vi "Do.vi"(6 "Input":variant, 8 "error in":errorcluster, 9 "Self Enqueuer":refnum<class "Message Enqueuer.lvclass">, 10 "Series Enqueuer":refnum<class "Message Enqueuer.lvclass">, 11 "Sample Watertemp PWM Control in":refnum<class "Sample Watertemp PWM Control.lvclass">) -> (0 "error out":errorcluster, 3 "Sample Watertemp PWM Control out":refnum<class "Sample Watertemp PWM Control.lvclass">)   [LabVIEW 2023, in "Sample Watertemp PWM Control.lvclass"]
uses:
  Sample Watertemp PWM Control.lvclass
  Sample Watertemp PWM Control.lvclass/Sample Watertemp PWM Control.ctl
  Task/Task Base/Task Base.lvclass
  Measure and Stimulus Subsystems/Measure and Stimulus Subsystems.lvclass
  <vilib>/ActorFramework/Message Enqueuer/Message Enqueuer.lvclass
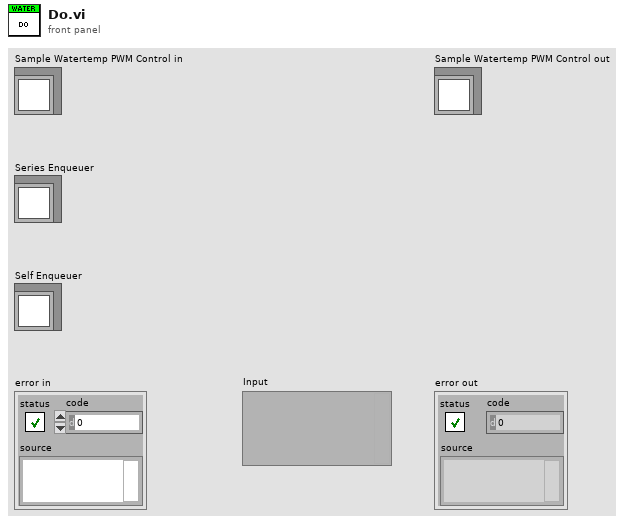
[diagram p1: front panel]
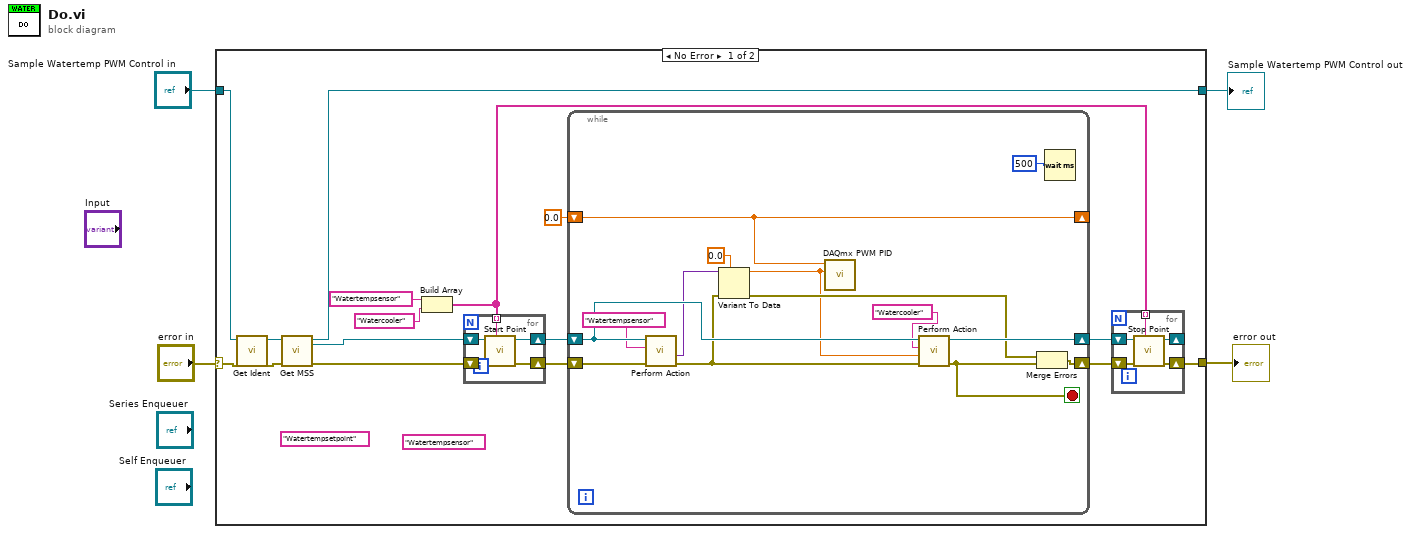
[diagram p0: block diagram]
diagram:
  n1 = case shown="No Error" "error in" {
    selector: "error in" -> [w5 w44]
    tunnel: [w13 w44] -> w1
    tunnel: [w9 w43] -> w4
    tunnel: "Sample Watertemp PWM Control in" -> [w7 w43]
    frame No Error {
      (unwired) "Watertempsetpoint" ("Target Name")
      (unwired) "Watertempsensor" ("Target Identifier")
      n2 = call "Get Ident.vi"("Task Base in"=w7) -> ("Task Base out"=w6:refnum<class "Sample Watertemp PWM Control.lvclass">)  [unwired: 9 in, 1 out]
      n3 = call "Get MSS.vi"("Task Base in"=w6) -> ("MSS"=w15:refnum<class "Measure and Stimulus Subsystems.lvclass">, "Task Base out"=w9:refnum<class "Sample Watertemp PWM Control.lvclass">)  [unwired: 9 in]
      n4 = Build Array("Watertempsensor" ("Target Identifier"), "Watercooler" ("Target Identifier")) -> (w10:string[])
      n5 = for {
        shift-right: [w23] -> w18
        shift-left: w5 -> [w21]
        shift-right: [w22] -> w17
        shift-left: w15 -> [w20]
        tunnel: w10 -> [w19] mode=indexing
        n6 = call "Start Point.vi"("Point Ident"=w19, "error in"=w21, "MSS in"=w20) -> ("error out"=w23:errorcluster, "MSS out"=w22:refnum<class "Measure and Stimulus Subsystems.lvclass">)  [unwired: 7 in]
      }
      n7 = while {
        shift-right: [w33] -> w16
        shift-left: w18 -> [w35]
        shift-right: [w36] -> w14
        shift-left: w17 -> [w34]
        shift-right: [w30] -> _
        shift-left: 0.0 -> [w30]
        stop <- w29 stop-if-true
        n8 = call "Perform Action.vi"("error in"=w35, "Point Ident"="Watertempsensor" ("Target Identifier"), "MSS in"=w34) -> ("error out"=w31:errorcluster, "Output"=w24:variant)  [unwired: 5 in, 2 out]
        n9 = Variant To Data(error in=w31, type=0.0, Variant=w24) -> (data=w26:dbl, error out=w28:errorcluster)
        n10 = call "DAQmx PWM PID.vi"("Process Variable"=w26, "Setpoint"=w30) -> ()  [unwired: 9 in, 1 out]
        n11 = call "Perform Action.vi"("error in"=w31, "Input"=w26, "Point Ident"="Watercooler" ("Target Ident"), "MSS in"=w34) -> ("error out"=w29:errorcluster, "MSS out"=w36:refnum<class "Measure and Stimulus Subsystems.lvclass">)  [unwired: 4 in, 2 out]
        n12 = Merge Errors(w28, w29) -> (w33:errorcluster)
        n13 = Wait (ms)(milliseconds to wait=u32 500) -> ()  [unwired: 1 out]
      }
      n14 = for {
        shift-right: [w40] -> w13
        shift-left: w16 -> [w42]
        tunnel: w10 -> [w38] mode=indexing
        shift-right: [w39] -> _
        shift-left: w14 -> [w41]
        n15 = call "Stop Point.vi"("Point Ident"=w38, "error in"=w42, "MSS in"=w41) -> ("error out"=w40:errorcluster, "MSS out"=w39:refnum<class "Measure and Stimulus Subsystems.lvclass">)  [unwired: 7 in]
      }
    }
    frame Error {
    }
  }
  "error out" <- w1
  "Sample Watertemp PWM Control out" <- w4
